vi "Initialize.vi"(8 "error in":errorcluster, 10 "parameters":variant, 11 "FPGA Instrument in":refnum<class "FPGA Instrument.lvclass">) -> (0 "error out":errorcluster, 2 "summary":T2[](array[typedef]), 3 "data value reference":T1)   [LabVIEW 2025, in "FPGA.lvlib" / "FPGA Instrument.lvclass"]
doc: "Initializes the data of a node to its default state.\nThe object is not created inside of this VI, because it is created from a File depending on user selection.\nCopyright 2017 National Instruments Corporation\n\nLicensed under the Apache License, Version 2.0 (the \"License\"); you may not use this file except in compliance with the License. You may obtain a copy of the License at http://www.apache.org/licenses/LICENSE-2.0\nUnless required by applicable law or agreed to in writing, software distributed under the License is distributed on an \"AS IS\" BASIS, WITHOUT WARRANTIES OR CONDITIONS OF ANY KIND, either express or implied. See the License for the specific language governing permissions and limitations under the License."
uses:
  FPGA Instrument.lvclass
  FPGA Instrument.lvclass/FPGA Instrument.ctl
  Users/Public/Documents/Sandia National Labs/TSS Plugin/CEF.lvlibp/Node/CEF_Node.lvclass
  Users/Public/Documents/Sandia National Labs/TSS Plugin/Abstract Engine.lvlibp/Plugin/Abstract/Abstract Instrument/Abstract Instrument.lvclass
  FPGA configuration/FPGA configuration.lvclass
  Users/Public/Documents/Sandia National Labs/TSS Plugin/CEF.lvlibp/Node/NodeRef.ctl
  Users/Public/Documents/Sandia National Labs/TSS Plugin/CEF.lvlibp/Node/Summary.ctl
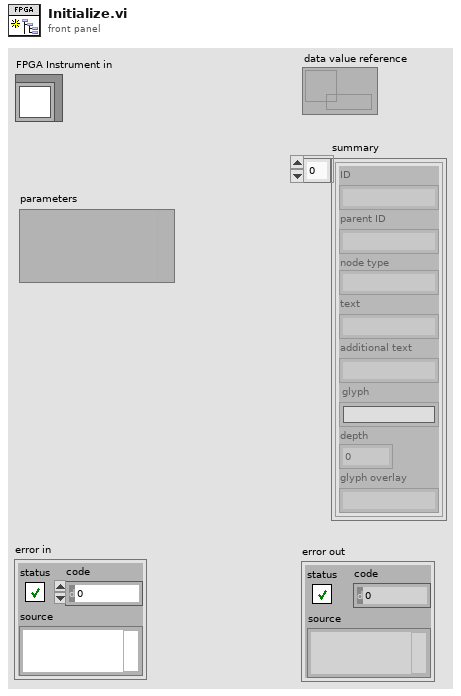
[diagram p1: front panel]
types:
  T1 = typedef "CEF.lvlibp/CEF_Node.lvclass/NodeRef.ctl" = refnum<data-value>
  T2 = typedef "CEF.lvlibp/CEF_Node.lvclass/Summary.ctl" = cluster{"ID":string, "parent ID":string, "node type":string, "text":string, "additional text":string, "glyph":string, "depth":i32, "glyph overlay":string}
  T3 = cluster{"Type":string, "Address":string, "SW Alias":string, "Description":string, "Enabled":bool}
  T4 = cluster{"ID":string, "parent ID":string, "node type":string, "text":string, "additional text":string, "glyph":string, "depth":i32, "glyph overlay":string}[]
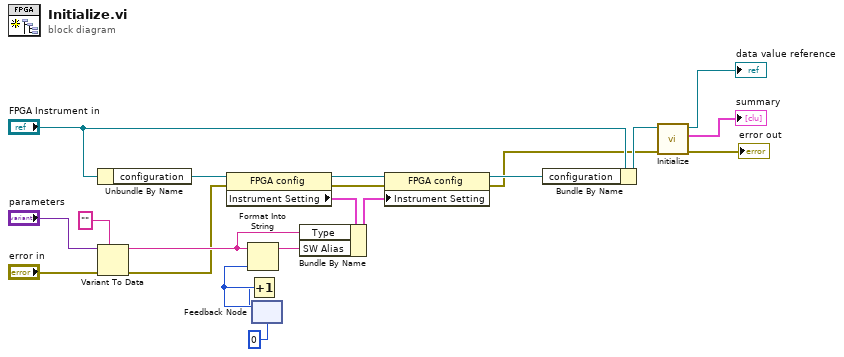
[diagram p0: block diagram]
diagram:
  n1 = Unbundle By Name("FPGA Instrument in") -> ("configuration"=w8:refnum<class "FPGA configuration.lvclass">)
  n2 = Variant To Data(error in="error in", type="", Variant="parameters") -> (data=w14:string, error out=w9:errorcluster)
  n3 = property class="FPGA config"(reference=w8, error in=w9) -> (reference out=w7:refnum<class "FPGA configuration.lvclass">, error out=w3:errorcluster, "Instrument Setting"=w5:T3)
  n4 = feedback #1(0) -> (w12:i32)
  n5 = Format Into String(initial string=w14, w12) -> (resulting string=w6:string)  [unwired: 2 in, 1 out]
  n6 = Increment(x=w12) -> (x+1=w11:i32)
  n7 = feedback-in #1(w11) -> ()
  n8 = Bundle By Name(cluster=w5, "Type"=w14, "SW Alias"=w6) -> (w4:T3)
  n9 = property class="FPGA config"(reference=w7, error in=w3, "Instrument Setting"=w4) -> (reference out=w16:refnum<class "FPGA configuration.lvclass">, error out=w2:errorcluster)
  n10 = Bundle By Name(cluster="FPGA Instrument in", "configuration"=w16) -> (w17:refnum<class "FPGA Instrument.lvclass">)
  n11 = call-parent "Initialize.vi"("error in"=w2, "CEF_Serialize node in"=w17) -> ("error out"=→"error out":errorcluster, "summary"=→"summary":T4, "data value reference"=→"data value reference":refnum<data-value>)  [unwired: 7 in]
